vi "Should Swap.vi"(9 "Person B":T1={"ID"=0, "Family Name"="Doe", "Given Name"="John", "Birth Date"=timestamp(3533142714.9178333 s since 1904-01-01)} {"Birth Date" format="%<%Y/%b/%d>T"}, 10 "Person A":T1={"ID"=0, "Family Name"="Smith", "Given Name"="John", "Birth Date"=timestamp(3533056306.0488334 s since 1904-01-01)} {"Birth Date" format="%<%Y/%b/%d>T"}, 11 "Swapper For Priority Month in":refnum<class "Swapper For Priority Month.lvclass">) -> (2 "Swap?":bool)   [LabVIEW 2023, in "Swapper For Priority Month.lvclass"]
uses:
  Swapper For Priority Month.lvclass
  Person Information.ctl
  Swapper For Priority Month.lvclass/Swapper For Priority Month.ctl
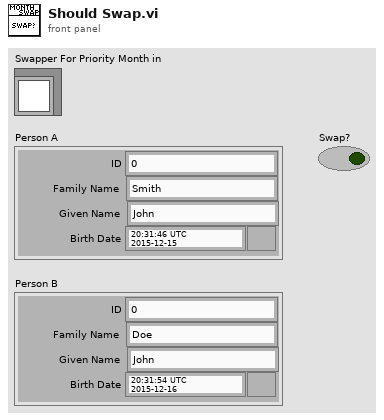
[diagram p1: front panel]
types:
  T1 = typedef "Person Information.ctl" = cluster{"ID":u32, "Family Name":string, "Given Name":string, "Birth Date":timestamp}
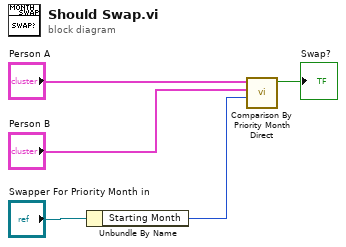
[diagram p0: block diagram]
diagram:
  n1 = Unbundle By Name("Swapper For Priority Month in") -> ("Starting Month"=w1:u32)
  n2 = call "Comparison By Priority Month Direct.vi"("Starting Month"=w1, "Person B"="Person B", "Person A"="Person A") -> ("Swap?"=→"Swap?":bool)  [unwired: 8 in]
